vi "Graph2D.vi"(0 "Experiment3D in":refnum<class "Experiment3D.lvclass">, 11 "error in (no error)":errorcluster) -> (4 "Experiment3D out":refnum<class "Experiment3D.lvclass">, 6 "X-2D":dbl[](array[numeric]), 8 "Y-2D":dbl[](array[numeric]), 15 "error out":errorcluster)   [LabVIEW 2014, in "Experiment3D.lvclass"]
uses:
  Experiment3D.lvclass
  Data/Data3D/Data3D.lvclass
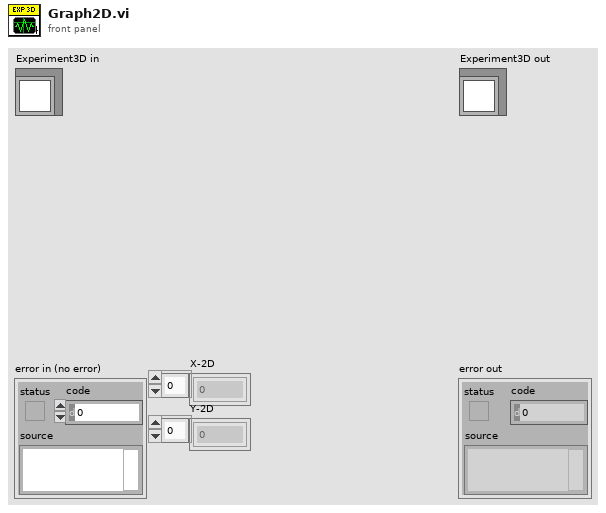
[diagram p1: front panel]
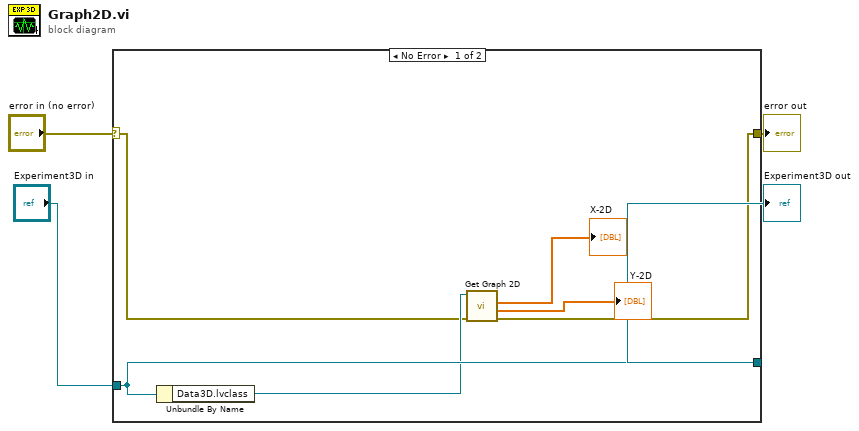
[diagram p0: block diagram]
diagram:
  n1 = case shown="No Error" "error in (no error)" {
    selector: "error in (no error)" -> [w7 w12]
    tunnel: [w8 w12] -> w3
    tunnel: [w10 w11] -> w1
    tunnel: "Experiment3D in" -> [w10 w11]
    frame No Error {
      n2 = Unbundle By Name(w10) -> ("Data3D.lvclass"=w9:refnum<class "Data3D.lvclass">)
      n3 = call "Get Graph 2D.vi"("error in (no error)"=w7, "Data3D in"=w9) -> ("error out"=w8:errorcluster, "Y-2D"=→"Y-2D":dbl[], "X-2D"=→"X-2D":dbl[])  [unwired: 6 in, 1 out]
    }
    frame Error {
    }
  }
  "error out" <- w3
  "Experiment3D out" <- w1
